vi "GetTemperatureAtHeight.vi"(7 "height":dbl, 10 "tank":T1, 11 "liquid":T2) -> (3 "temperature":dbl)   [LabVIEW 2020]
doc: "Returns the temperature at point in the simulation closes to the required height, at the wall of the tank."
uses:
  Liquid.ctl
  TankResolution.ctl
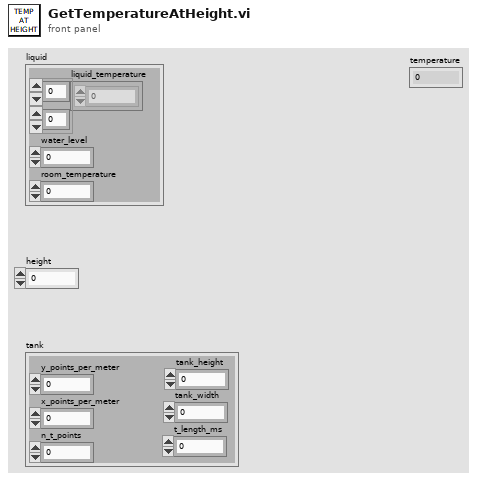
[diagram p1: front panel]
types:
  T1 = typedef "TankResolution.ctl" = cluster{"y_points_per_meter":i32, "x_points_per_meter":i32, "n_t_points":i32, "tank_height":dbl, "tank_width":dbl, "t_length_ms":u32}
  T2 = typedef "Liquid.ctl" = cluster{"liquid_temperature":dbl[][], "water_level":dbl, "room_temperature":dbl}
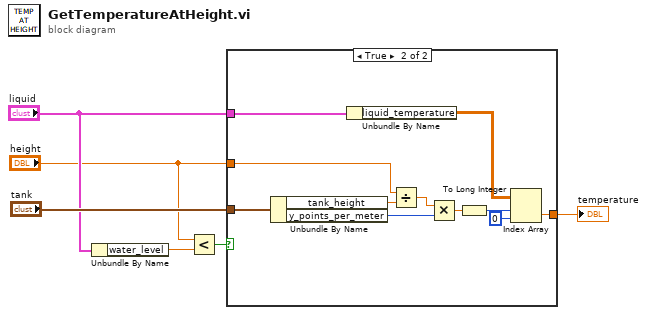
[diagram p0: block diagram]
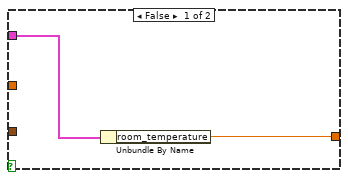
[diagram p2: hidden frame]
diagram:
  n1 = Unbundle By Name("liquid") -> ("water_level"=w2:dbl)
  n2 = Less?(x="height", y=w2) -> (x < y?=w3:bool)
  n3 = case shown="True" w3 {
    tunnel: [w7 w19] -> w6
    tunnel: "liquid" -> [w8 w16]
    tunnel: "tank" -> [_ w14]
    tunnel: "height" -> [_ w10]
    frame False {
      n4 = Unbundle By Name(w8) -> ("room_temperature"=w7:dbl)
    }
    frame True {
      n5 = Unbundle By Name(w14) -> ("tank_height"=w9:dbl, "y_points_per_meter"=w12:i32)
      n6 = Unbundle By Name(w16) -> ("liquid_temperature"=w17:dbl[][])
      n7 = Divide(x=w10, y=w9) -> (x/y=w11:dbl)
      n8 = Multiply(x=w11, y=w12) -> (x*y=w13:dbl)
      n9 = To Long Integer(number=w13) -> (32bit integer=w15:i32)
      n10 = Index Array(array=w17, index (row)=w15, index (col)=0 ("index")) -> (element=w19:dbl)
    }
  }
  "temperature" <- w6
